vi "DB Tools Get DB From Provider.vi"(4 "DBMS Name":string, 7 "Provider":string) -> (3 "database":T1)   [LabVIEW 2017, in "NI_Database_API.lvlib"]
doc: "Specifies the type of database given the OLE DB provider name and the DBMS name."
uses:
  <vilib>/addons/database/NI_Database_API.lvlib
  <vilib>/addons/database/Auxilliary.llb/DB Tools Database.ctl
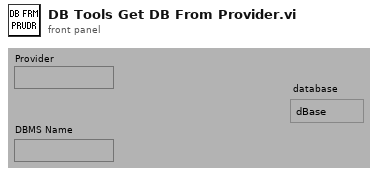
[diagram p1: front panel]
types:
  T1 = typedef "NI_Database_API.lvlib/DB Tools Database.ctl" = enum16{"dBase", "Jet", "SQL Server", "Oracle", "MySql"}
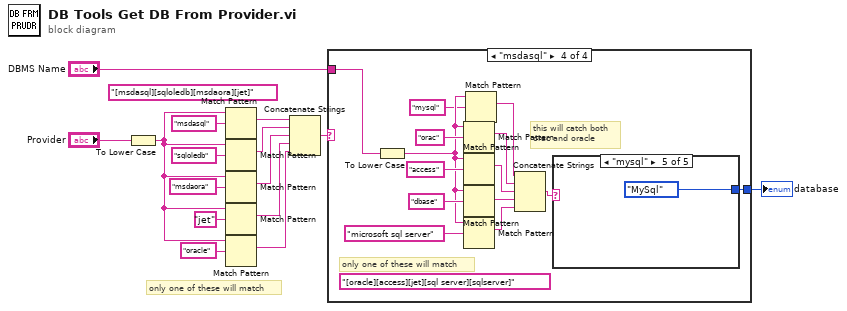
[diagram p0: block diagram]
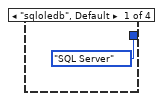
[diagram p2: hidden frame]
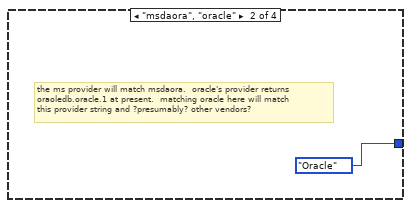
[diagram p3: hidden frame]
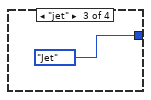
[diagram p4: hidden frame]
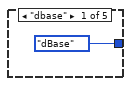
[diagram p5: hidden frame]
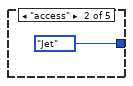
[diagram p6: hidden frame]
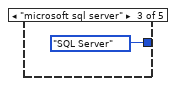
[diagram p7: hidden frame]
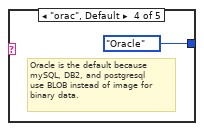
[diagram p8: hidden frame]
diagram:
  (unwired) "[msdasql][sqloledb][msdaora][jet]" ("regular expression")
  # "only one of these will match"
  n1 = To Lower Case(string="Provider") -> (all lower case string=w4:string)
  n2 = Match Pattern(string=w4, regular expression="msdasql") -> (match substring=w11:string)  [unwired: 1 in, 3 out]
  n3 = Match Pattern(string=w4, regular expression="sqloledb") -> (match substring=w7:string)  [unwired: 1 in, 3 out]
  n4 = Match Pattern(string=w4, regular expression="msdaora") -> (match substring=w10:string)  [unwired: 1 in, 3 out]
  n5 = Match Pattern(string=w4, regular expression="jet") -> (match substring=w9:string)  [unwired: 1 in, 3 out]
  n6 = Match Pattern(string=w4, regular expression="oracle" ("string")) -> (match substring=w3:string)  [unwired: 1 in, 3 out]
  n7 = Concatenate Strings(w11, w7, w10, w9, w3) -> (w8:string)
  n8 = case shown="\"msdasql\"" w8 {
    tunnel: [DB_Tools_Database."SQL Server" ("database") DB_Tools_Database."Oracle" ("database") DB_Tools_Database."Jet" ("database") w32] -> w2
    tunnel: "DBMS Name" -> [_ _ _ w22]
    frame "sqloledb", Default {
    }
    frame "msdaora", "oracle" {
      # "the ms provider will match msdaora.  oracle's provider returns\noraoledb.oracle.1 at present.  matching oracle here will match\nthis provider string and ?presumably? other vendors?"
    }
    frame "jet" {
    }
    frame "msdasql" {
      (unwired) "[oracle][access][jet][sql server][sqlserver]" ("string")
      # "this will catch both\norac and oracle"
      # "only one of these will match"
      n9 = To Lower Case(string=w22) -> (all lower case string=w20:string)
      n10 = Match Pattern(string=w20, regular expression="orac") -> (match substring=w27:string)  [unwired: 1 in, 3 out]
      n11 = Match Pattern(string=w20, regular expression="access") -> (match substring=w26:string)  [unwired: 1 in, 3 out]
      n12 = Match Pattern(string=w20, regular expression="dbase") -> (match substring=w25:string)  [unwired: 1 in, 3 out]
      n13 = Match Pattern(string=w20, regular expression="microsoft sql server") -> (match substring=w24:string)  [unwired: 1 in, 3 out]
      n14 = Match Pattern(string=w20, regular expression="mysql") -> (match substring=w21:string)  [unwired: 1 in, 3 out]
      n15 = Concatenate Strings(w21, w27, w26, w25, w24) -> (w28:string)
      n16 = case shown="\"mysql\"" w28 {
        tunnel: [DB_Tools_Database."dBase" ("database") DB_Tools_Database."Jet" ("database") DB_Tools_Database."SQL Server" ("database") DB_Tools_Database."Oracle" ("database") DB_Tools_Database."MySql" ("database")] -> w32
        frame "dbase" {
        }
        frame "access" {
        }
        frame "microsoft sql server" {
        }
        frame "orac", Default {
          # "Oracle is the default because\nmySQL, DB2, and postgresql \nuse BLOB instead of image for\nbinary data."
        }
        frame "mysql" {
        }
      }
    }
  }
  "database" <- w2
